vi "Configure Modulation (PWM).vi"(0 "VISA resource name":refnum<visa-resource-name>, 1 "Modulation Waveform (0: Sine)":u16(ring) items=["Sine", "Square", "Triangle", "UpRamp", "DnRamp", "Noise", "Arb"], 2 "Modulation Frequency (100 Hz)":dbl=100.0, 5 "Channel (1: Channel 1)":i32(ring)=1 items=["Channel 1"=1, "Channel 2"=2], 7 "Enable Pulse Width Modulation (T:Enable)":bool=TRUE, 9 "PWM Source (0: Internal)":u16(ring) items=["Internal", "External"], 11 "error in (no error)":errorcluster, 12 "Pulse Width (0.0002 s)":dbl=0.0002) -> (4 "VISA resource name out":refnum<visa-resource-name>, 15 "error out":errorcluster)   [LabVIEW 2023, in "Siglent SDG X Series.lvlib"]
doc: "Configures and enables FSK modulation.\n\nNote: PWM modulation is only available for Pulse waveform."
uses:
  Siglent SDG X Series.lvlib
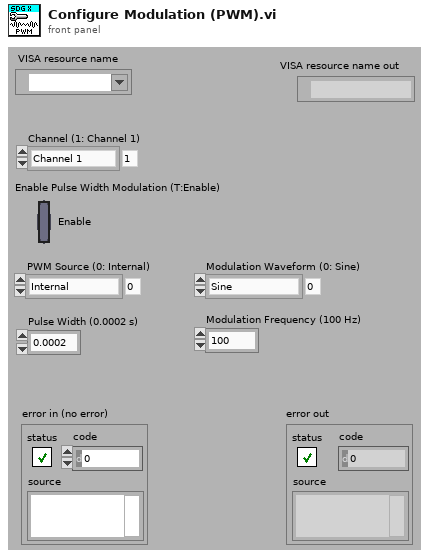
[diagram p1: front panel]
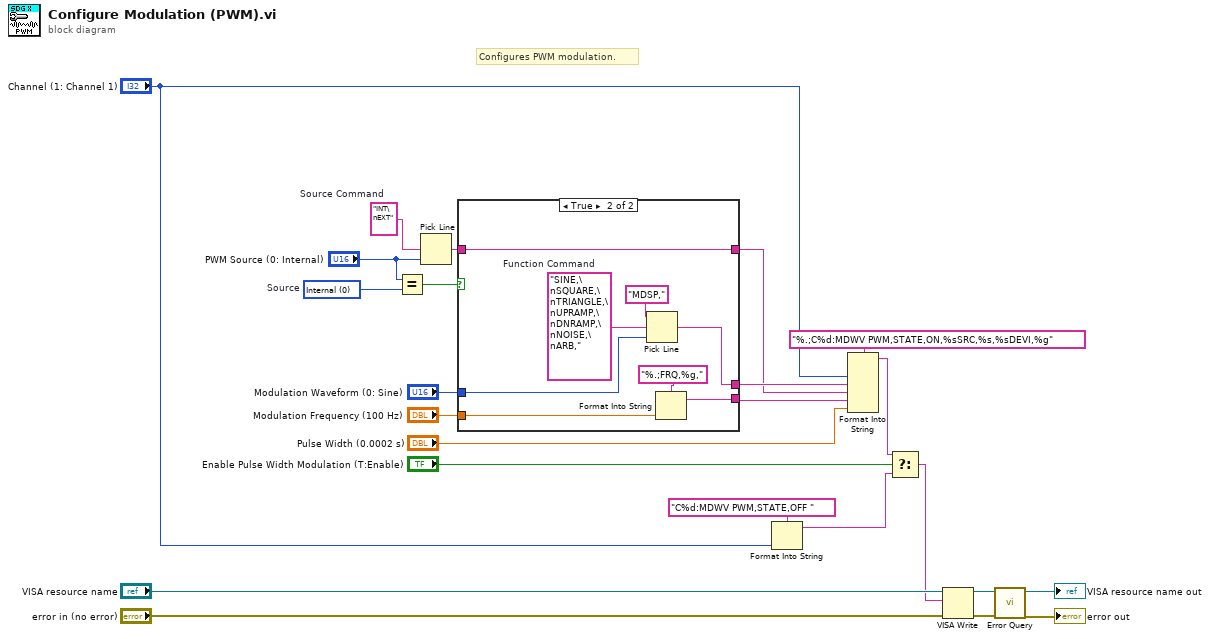
[diagram p0: block diagram]
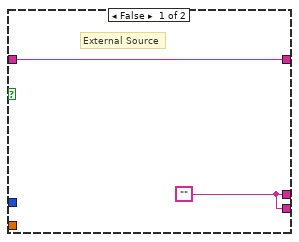
[diagram p2: hidden frame]
diagram:
  w14 = u16 0 items=["Internal", "External"]  # Source
  w15 = "INT\nEXT"  # Source Command
  # "Configures PWM modulation."
  n1 = Equal?(x="PWM Source (0: Internal)", y=w14) -> (x = y?=w13:bool)
  n2 = Pick Line(multi-line string=w15, line index="PWM Source (0: Internal)") -> (output string=w12:string)  [unwired: 1 in]
  n3 = case shown="True" w13 {
    tunnel: w12 -> [w26 w32]
    tunnel: "Modulation Waveform (0: Sine)" -> [_ w33]
    tunnel: "Modulation Frequency (100 Hz)" -> [_ w29]
    tunnel: [w26 w32] -> w9
    tunnel: [w25 w30] -> w10
    tunnel: [w25 w27] -> w8
    frame False {
      w25 = ""
      # "External Source"
    }
    frame True {
      w34 = "SINE,\nSQUARE,\nTRIANGLE,\nUPRAMP,\nDNRAMP,\nNOISE,\nARB,"  # Function Command
      n4 = Pick Line(string ("")="MDSP,", multi-line string=w34, line index=w33) -> (output string=w30:string)
      n5 = Format Into String(format string="%.;FRQ,%g,", w29) -> (resulting string=w27:string)  [unwired: 2 in, 1 out]
    }
  }
  n6 = Format Into String(format string="C%d:MDWV PWM,STATE,OFF ", "Channel (1: Channel 1)") -> (resulting string=w4:string)  [unwired: 2 in, 1 out]
  n7 = Format Into String(format string="%.;C%d:MDWV PWM,STATE,ON,%sSRC,%s,%sDEVI,%g", "Channel (1: Channel 1)", w10, w9, w8, "Pulse Width (0.0002 s)") -> (resulting string=w6:string)  [unwired: 2 in, 1 out]
  n8 = Select(t=w6, s="Enable Pulse Width Modulation (T:Enable)", f=w4) -> (s? t:f=w1:string)
  n9 = VISA Write(VISA resource name="VISA resource name", write buffer=w1, error in (no error)="error in (no error)") -> (VISA resource name out=w22:refnum<visa-resource-name>, error out=w21:errorcluster)  [unwired: 1 out]
  n10 = call "Error Query.vi"("error in (no error)"=w21, "VISA resource name"=w22) -> ("error out"=→"error out":errorcluster, "VISA resource name out"=→"VISA resource name out":refnum<visa-resource-name>)  [unwired: 6 in, 2 out]
